vi "Verify Response.vi"(8 "error in (no error)":errorcluster, 9 "timeout ms (25000)":i32=25000, 10 "Message":string, 11 "Sift Client in":refnum<class "Sift Client.lvclass">) -> (0 "error out":errorcluster, 2 "data":variant, 3 "Sift Client out":refnum<class "Sift Client.lvclass">)   [LabVIEW 2024, in "Sift Client.lvlib" / "Sift Client.lvclass"]
uses:
  Sift Client.lvclass
  Sift Client.lvclass/Sift Client.ctl
  <userlib>/_OpenG.lib/error/error.llb/openg_error.lvlib
  <vilib>/addons/_JKI.lib/Serialization/JSON/JKI JSON Serialization.lvlib
  <vilib>/ErrorRing/Error Ring.xnode
  <vilib>/Utility/error.llb/Error Cluster From Error Code.vi
  Private/Typedefs/Messages/JSON Response.ctl
  Sift Client.lvlib
  Private/Typedefs/Messages/Reason.ctl
panel:
  out "Response Data":string
  out "Message Size":u32
  out "Message Type":u8
  in  "Reason":T1
  in  "JSON Response":T2
  out "Response Header":string
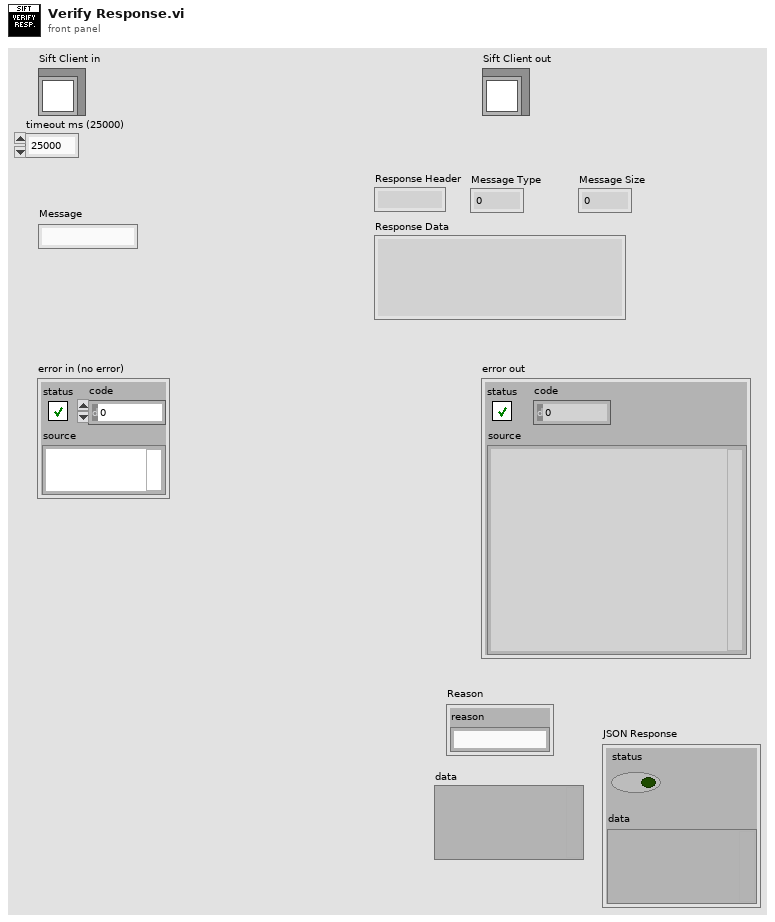
[diagram p1: front panel]
types:
  T1 = typedef "Sift Client.lvlib/Reason.ctl" = cluster{"reason":string}
  T2 = typedef "Sift Client.lvlib/JSON Response.ctl" = cluster{"status":bool, "data":variant}
  T3 = enum16{"Standard", "Buffered", "CRLF", "Immediate"}
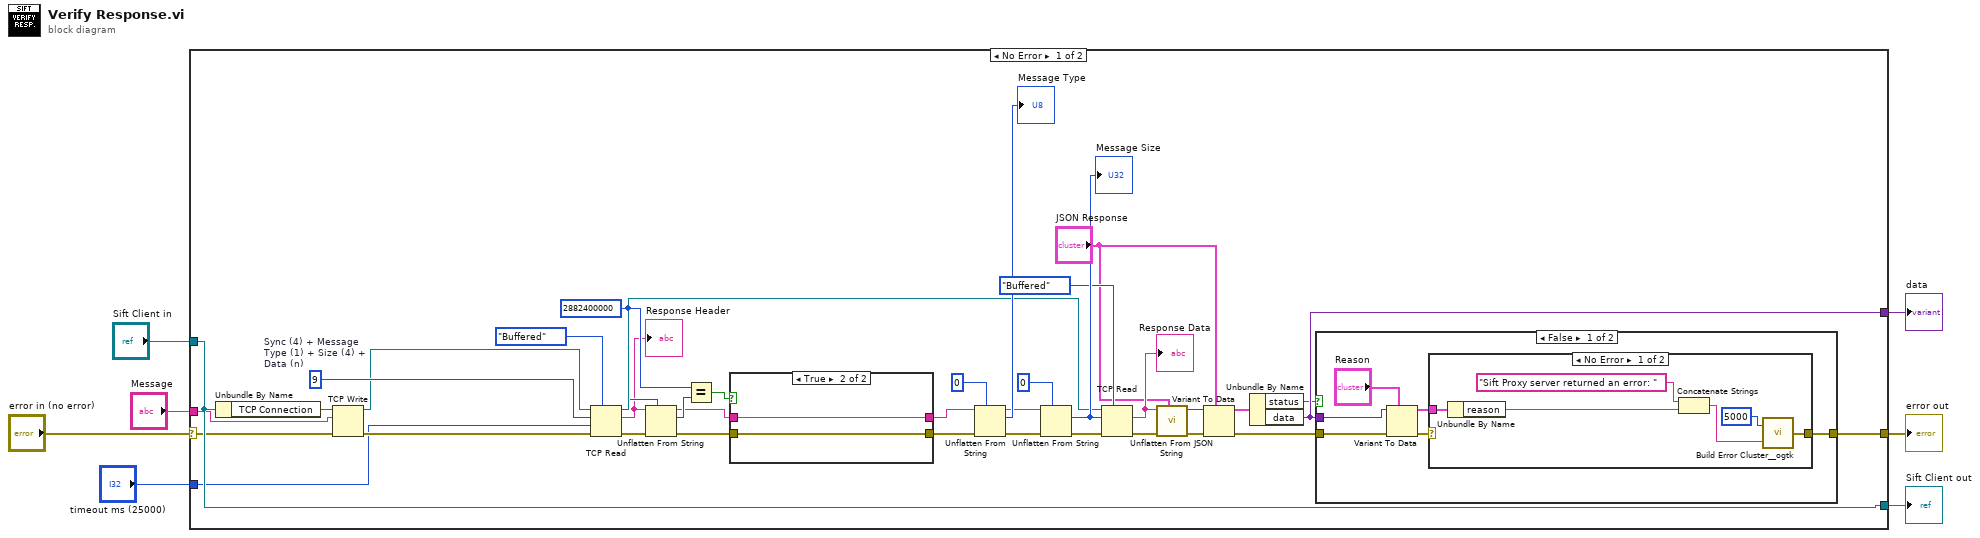
[diagram p0: block diagram]
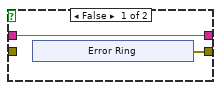
[diagram p2: hidden frame]
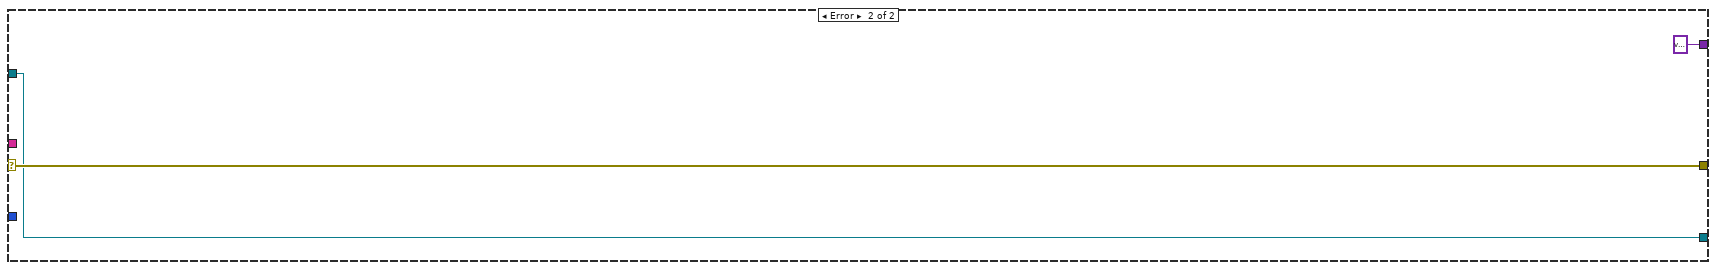
[diagram p5: hidden frame]
diagram:
  n1 = case shown="No Error" "error in (no error)" {
    selector: "error in (no error)" -> [w12 w70]
    tunnel: [w42 w70] -> w6
    tunnel: [w43 w69] -> w4
    tunnel: "Sift Client in" -> [w43 w69]
    tunnel: [w41 variant ("data")] -> w3
    tunnel: "Message" -> [w13 _]
    tunnel: "timeout ms (25000)" -> [w8 _]
    frame No Error {
      w22 = u32 2882400000
      w40 = 9  # Sync (4) + Message Type (1) + Size (4) + Data (n)
      n2 = Unbundle By Name(w43) -> ("TCP Connection"=w10:refnum<k5>)
      n3 = TCP Write(connection ID=w10, data in=w13, error in (no error)=w12) -> (connection ID out=w9:refnum<k5>, error out=w11:errorcluster)  [unwired: 1 in, 1 out]
      n4 = TCP Read(connection ID=w9, bytes to read=w40, error in (no error)=w11, 7:T3."Buffered" ("mode (standard)"), 9:w8) -> (connection ID out=w30:refnum<k5>, data out=w18:string, error out=w24:errorcluster)
      "Response Header" <- w18
      n5 = Unflatten From String(type=w22, binary string=w18, error in (no error)=w24) -> (rest of the binary string=w16:string, value=w23:u32, error out=w19:errorcluster)  [unwired: 2 in]
      n6 = Equal?(x=w22, y=w23) -> (x = y?=w21:bool)
      n7 = case shown="True" w21 {
        tunnel: [w46 w53] -> w20
        tunnel: w19 -> [_ w53]
        tunnel: [w45 w52] -> w17
        tunnel: w16 -> [w45 w52]
        frame False {
          n8 = xnode "Error Ring"() -> ("error out"=w46:errorcluster)
        }
        frame True {
        }
      }
      n9 = Unflatten From String(type=u8 0, binary string=w17, error in (no error)=w20) -> (rest of the binary string=w37:string, value=→"Message Type":u8, error out=w35:errorcluster)  [unwired: 2 in]
      n10 = Unflatten From String(type=u32 0, binary string=w37, error in (no error)=w35) -> (value=w32:u32, error out=w34:errorcluster)  [unwired: 2 in, 1 out]
      "Message Size" <- w32
      n11 = TCP Read(connection ID=w30, bytes to read=w32, error in (no error)=w34, 7:T3."Buffered" ("mode (standard)")) -> (data out=w29:string, error out=w33:errorcluster)  [unwired: 1 in, 1 out]
      "Response Data" <- w29
      n12 = call <vilib>:"Unflatten From JSON String.vi"("Type and Defaults"="JSON Response", "error in"=w33, "JSON String"=w29) -> ("error out"=w15:errorcluster, "Variant"=w26:variant)  [unwired: 7 in]
      n13 = Variant To Data(error in=w15, type="JSON Response", Variant=w26) -> (data=w27:T2, error out=w14:errorcluster)
      n14 = Unbundle By Name(w27) -> ("status"=w28:bool, "data"=w41:variant)
      n15 = case shown="False" w28 {
        tunnel: [w59 w67] -> w42
        tunnel: w14 -> [w55 w67]
        tunnel: w41 -> [w57 _]
        frame False {
          n16 = Variant To Data(error in=w55, type="Reason", Variant=w57) -> (data=w58:T1, error out=w54:errorcluster)
          n17 = case shown="No Error" w54 {
            selector: w54 -> [_ w66]
            tunnel: [w65 w66] -> w59
            tunnel: w58 -> [w63 _]
            frame No Error {
              n18 = Unbundle By Name(w63) -> ("reason"=w61:string)
              n19 = Concatenate Strings("Sift Proxy server returned an error: ", w61) -> (w60:string)
              n20 = call <userlib>:"Build Error Cluster__ogtk.vi"("String to Prepend to source (\"\")"=w60, "code"=5000) -> ("error out"=w65:errorcluster)
            }
            frame Error {
            }
          }
        }
        frame True {
        }
      }
    }
    frame Error {
    }
  }
  "error out" <- w6
  "Sift Client out" <- w4
  "data" <- w3
